vi "Read File.vi"(10 "MXN":bool, 11 "Coffee Actor in":refnum<class "Coffee Actor.lvclass">) -> (3 "Array":string[][](array[string]))   [LabVIEW 2019, in "Coffee Actor.lvlib" / "Coffee Actor.lvclass"]
uses:
  Coffee Actor.lvclass
  <vilib>/Utility/config.llb/Read Key (Double).vi
  <vilib>/Utility/config.llb/Read Key (String).vi
  <vilib>/Utility/config.llb/NI_LVConfig.lvlib
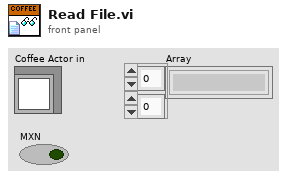
[diagram p1: front panel]
types:
  T1 = typedef "NI_LVConfig.lvlib/Config Data RefNum.ctl" = refnum<k1>
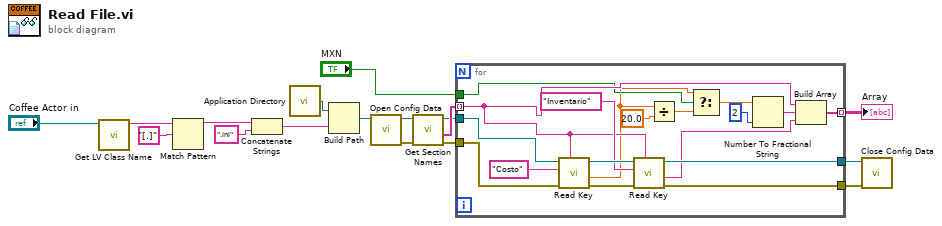
[diagram p0: block diagram]
diagram:
  n1 = call <vilib>:"Get LV Class Name.vi"("object"="Coffee Actor in") -> ("class name"=w7:string)  [unwired: 9 in, 1 out]
  n2 = Match Pattern(string=w7, regular expression="[.]") -> (before substring=w9:string)  [unwired: 1 in, 3 out]
  n3 = Concatenate Strings(w9, ".ini" ("string")) -> (w3:string)
  n4 = call <vilib>:"Application Directory.vi"() -> ("Application Directory"=w1:path)
  n5 = Build Path(base path=w1, name or relative path=w3) -> (appended path=w4:path)
  n6 = call <vilib>:"Open Config Data.vi"("configuration file path"=w4) -> ("error out"=w12:errorcluster, "refnum"=w10:T1)  [unwired: 8 in, 1 out]
  n7 = call <vilib>:"Get Section Names.vi"("error in (no error)"=w12, "refnum"=w10) -> ("error out"=w13:errorcluster, "section names"=w14:string[], "refnum out"=w11:T1)  [unwired: 7 in]
  n8 = for {
    tunnel: w11 -> [w34]
    tunnel: w13 -> [w35]
    tunnel: [w31] -> w5
    tunnel: [w30] -> w6
    tunnel: w14 -> [w27] mode=indexing
    tunnel: [w25] -> w15 mode=indexing
    tunnel: "MXN" -> [w22]
    n9 = call-poly <vilib>:"Read Key.vi"("section"=w27, "error in (no error)"=w35, "key"="Costo" ("section"), "refnum"=w34) -> ("error out"=w33:errorcluster, "value"=w19:dbl, "refnum out"=w32:T1)  [unwired: 4 in, 1 out]
    n10 = call-poly <vilib>:"Read Key.vi"("section"=w27, "error in (no error)"=w33, "key"="Inventario" ("section"), "refnum"=w32) -> ("error out"=w31:errorcluster, "value"=w26:string, "refnum out"=w30:T1)  [unwired: 4 in, 1 out]
    n11 = Divide(x=w19, y=20.0) -> (x/y=w20:dbl)
    n12 = Select(t=w19, s=w22, f=w20) -> (s? t:f=w21:dbl)
    n13 = Number To Fractional String(number=w21, precision (6)=i16 2) -> (F-format string=w24:string)  [unwired: 2 in]
    n14 = Build Array(w27, w24, w26) -> (w25:string[])
  }
  "Array" <- w15
  n15 = call <vilib>:"Close Config Data.vi"("error in (no error)"=w5, "refnum"=w6) -> ()  [unwired: 8 in, 2 out]
